vi "File.Get List of Oversized Files.vi"(8 "error in (no error)":errorcluster, 10 "Max Size (MB)":dbl, 11 "RootDir":path) -> (0 "error out":errorcluster, 2 "OverSize Files":cluster{"Name":string, "Path":path, "MB":dbl}[](array[cluster]) {"MB" format="%.3f"}, 3 "Files":cluster{"Name":string, "Path":path, "MB":dbl}[](array[cluster]) {"MB" format="%.3f"})   [LabVIEW 2024]
uses:
  File Utils.lvlib
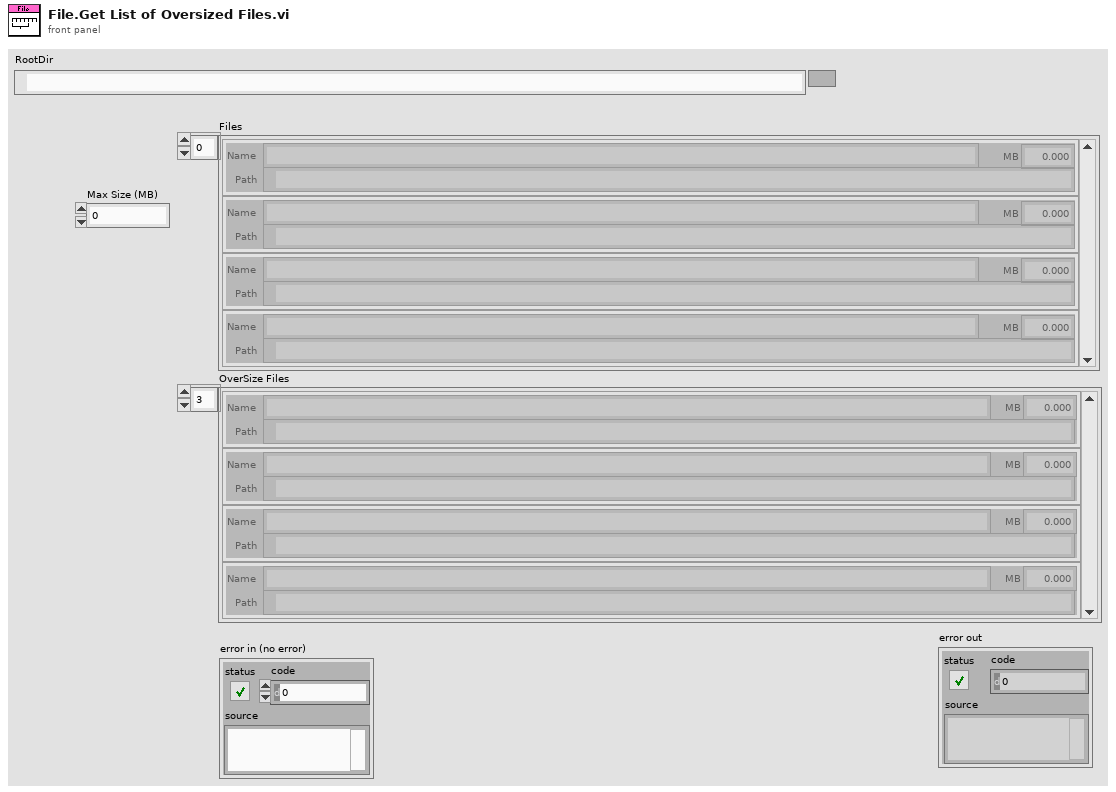
[diagram p1: front panel]
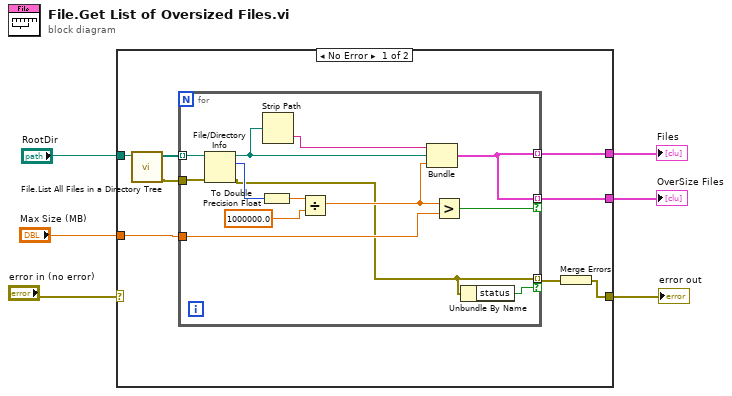
[diagram p0: block diagram]
diagram:
  n1 = case shown="No Error" "error in (no error)" {
    selector: "error in (no error)" -> [_ w28]
    tunnel: "RootDir" -> [w14 _]
    tunnel: [w12 _] -> w5
    tunnel: "Max Size (MB)" -> [w11 _]
    tunnel: [w10 _] -> w3
    tunnel: [w8 w28] -> w1
    frame No Error {
      n2 = call "File.List All Files in a Directory Tree.vi"("Folder"=w14) -> ("error out"=w9:errorcluster, "Files"=w13:path[])  [unwired: 9 in]
      n3 = for {
        tunnel: w13 -> [w27] mode=indexing
        tunnel: [w24] -> w12 mode=indexing
        tunnel: [w24] -> w10 mode=indexing if=w22
        tunnel: w11 -> [w23]
        tunnel: w9 -> [w17]
        tunnel: [w16] -> w7 mode=indexing if=w15
        n4 = File/Directory Info(path=w27, error in=w17) -> (path out=w25:path, size=w20:i64, error out=w16:errorcluster)  [unwired: 4 out]
        n5 = To Double Precision Float(number=w20) -> (double precision float=w21:dbl)
        n6 = Strip Path(path=w25) -> (name=w26:string)  [unwired: 1 out]
        n7 = Divide(x=w21, y=1000000.0) -> (x/y=w18:dbl)
        n8 = Bundle("name"=w26, "path out"=w25, w18) -> (w24:cluster{"name":string, "path out":path, dbl})  [unwired: 1 in]
        n9 = Greater?(x=w18, y=w23) -> (0:w22:bool)
        n10 = Unbundle By Name(w16) -> ("status"=w15:bool)
      }
      n11 = Merge Errors(w7) -> (w8:errorcluster)
    }
    frame Error {
    }
  }
  "Files" <- w5
  "OverSize Files" <- w3
  "error out" <- w1
